vi "Labview_USB_GPIO_Test.vi"() -> ()   [LabVIEW 2012]
uses:
  Ginkgo PWM/Labview_USB_PWM_Test/lib/labview_32bit/ControlGPIO/Ginkgo_Driver.dll
panel:
  out "error out":errorcluster
  in  "stop":bool
  out "P8":bool
  out "P9":bool
  out "P10":bool
  out "P11":bool
  out "P12":bool
  out "P13":bool
  out "P14":bool
  out "P15":bool
  in  "P7":bool
  in  "P6":bool
  in  "P5":bool
  in  "P4":bool
  in  "P3":bool
  in  "P2":bool
  in  "P1":bool
  in  "P0":bool
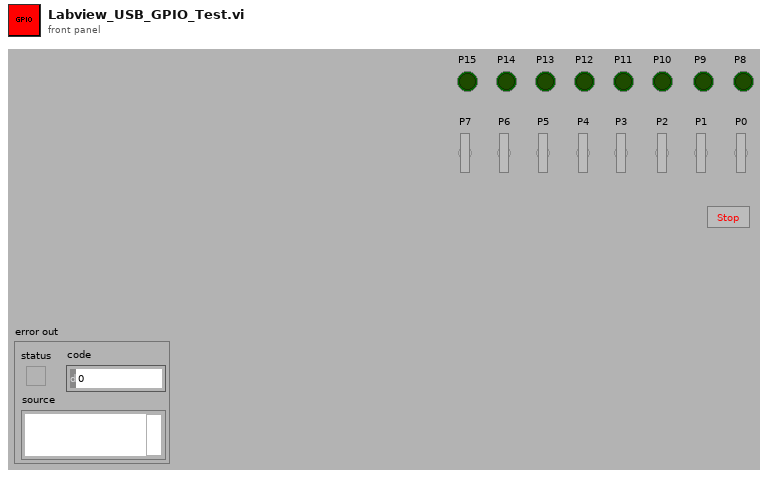
[diagram p1: front panel]
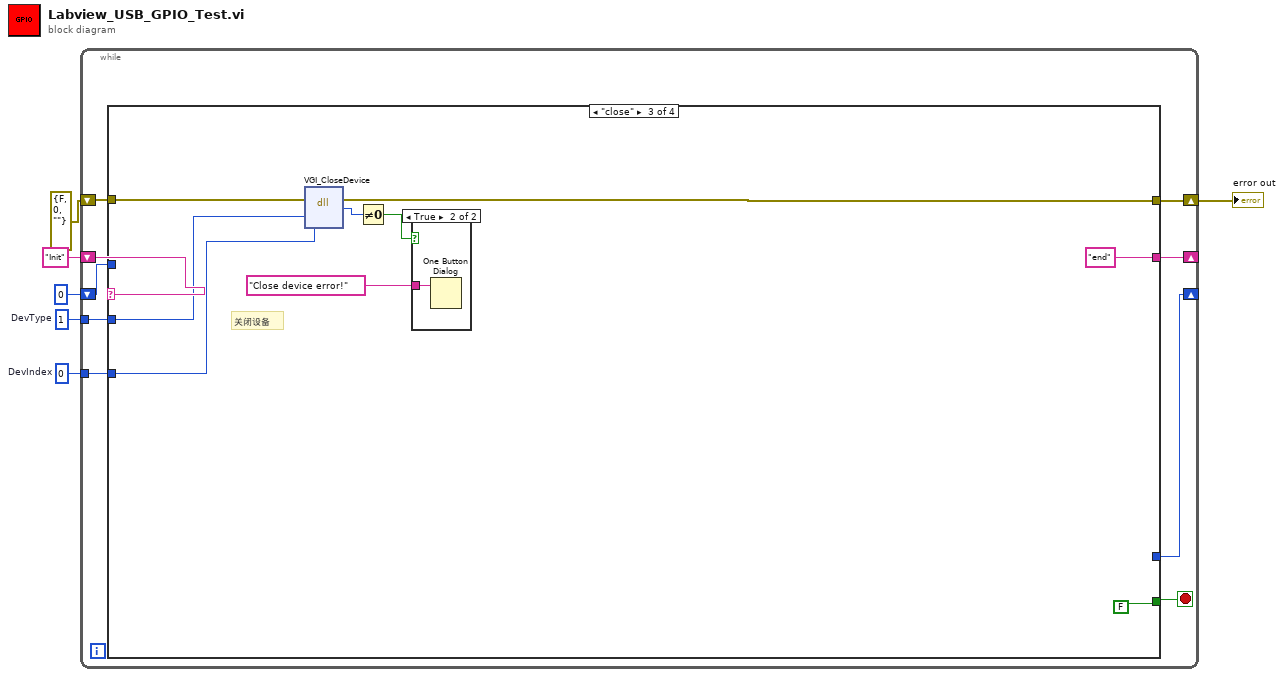
[diagram p0: block diagram]
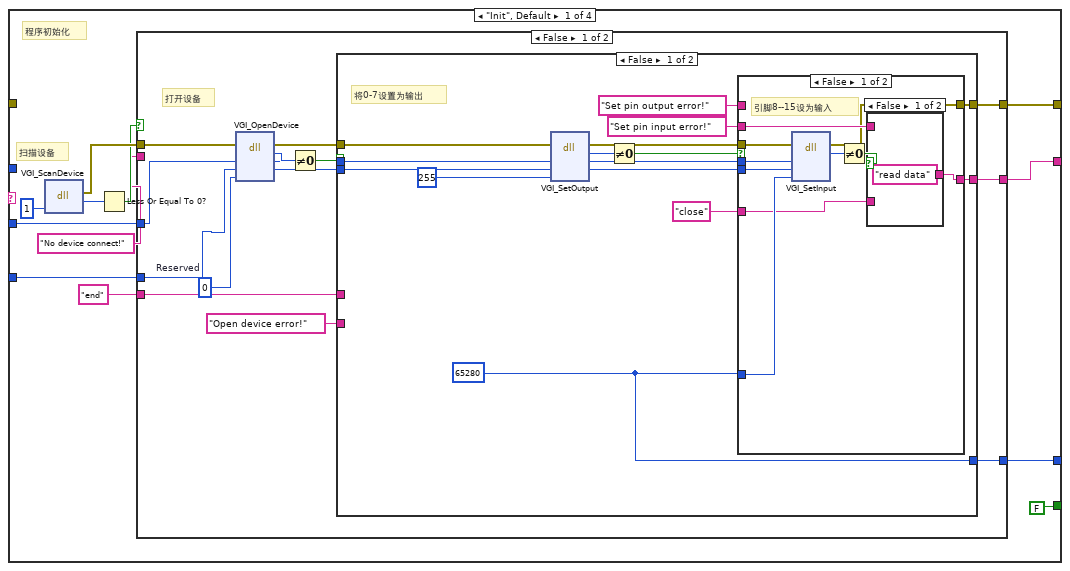
[diagram p2: hidden frame]
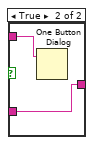
[diagram p3: hidden frame]
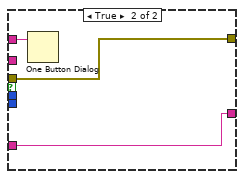
[diagram p4: hidden frame]
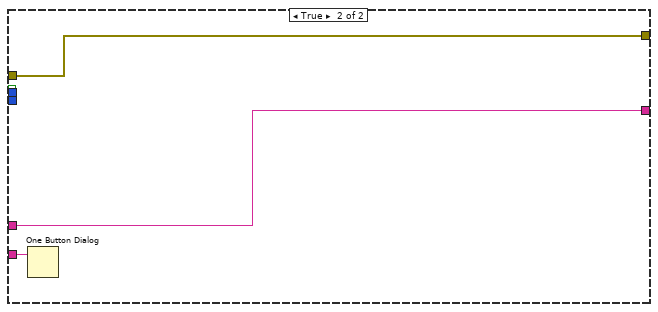
[diagram p5: hidden frame]
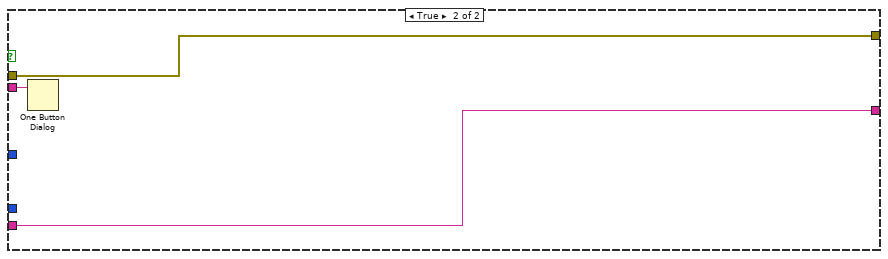
[diagram p6: hidden frame]
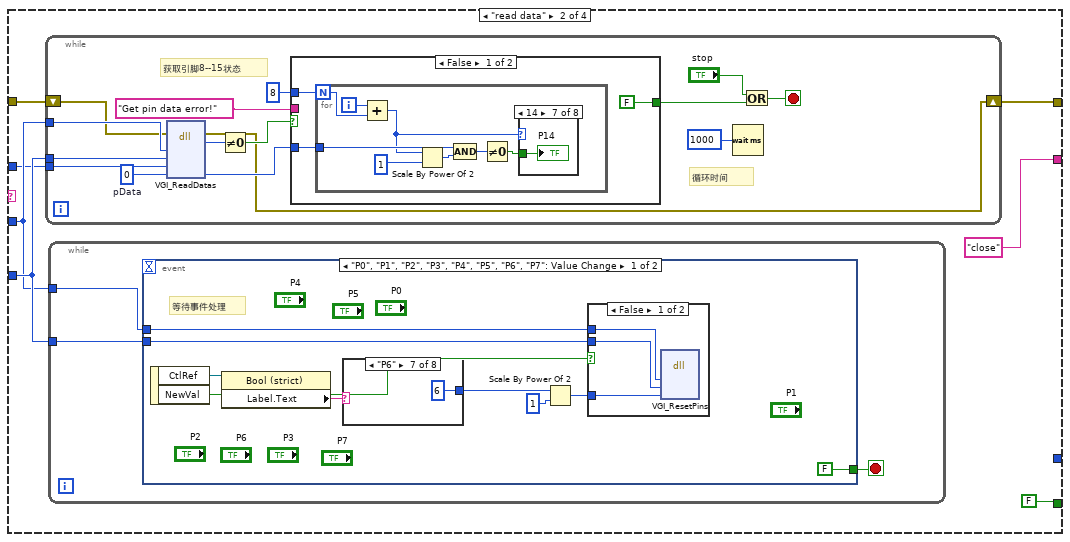
[diagram p7: hidden frame]
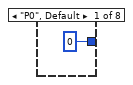
[diagram p8: hidden frame]
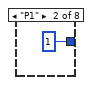
[diagram p9: hidden frame]
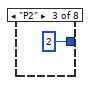
[diagram p10: hidden frame]
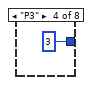
[diagram p11: hidden frame]
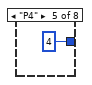
[diagram p12: hidden frame]
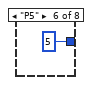
[diagram p13: hidden frame]
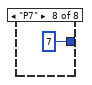
[diagram p14: hidden frame]
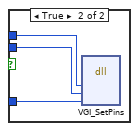
[diagram p15: hidden frame]
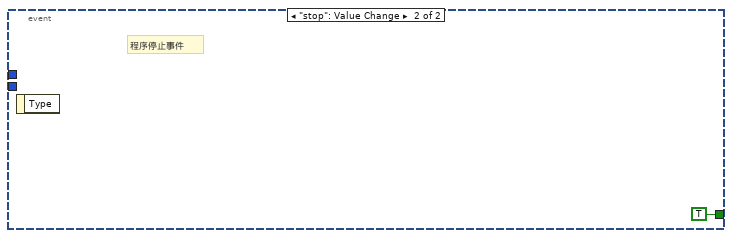
[diagram p16: hidden frame]
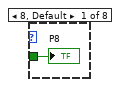
[diagram p17: hidden frame]
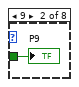
[diagram p18: hidden frame]
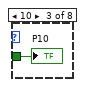
[diagram p19: hidden frame]
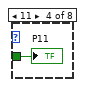
[diagram p20: hidden frame]
diagram:
  w4 = 0  # DevIndex
  w5 = 1  # DevType
  n1 = while {
    shift-right: [w14] -> _
    shift-left: "Init" -> [w15]
    tunnel: w5 -> [w13]
    tunnel: w4 -> [w12]
    shift-right: [w11] -> _
    shift-left: u16 0 -> [w10]
    shift-right: [w8] -> w2
    shift-left: errorcluster {"status"=FALSE, "code"=0, "source"=""} ("error out") -> [w7]
    stop <- w9 stop-if-true
    n2 = case shown="\"close\"" w15 {
      tunnel: [w21 "close" "end" "end"] -> w14
      tunnel: w13 -> [w20 w83 w149 _]
      tunnel: w12 -> [w19 w84 w150 _]
      tunnel: [w18 _ _ _] -> w11
      tunnel: w10 -> [_ w82 _ _]
      tunnel: [FALSE FALSE FALSE TRUE] -> w9
      tunnel: [w16 w79 w151 w159] -> w8
      tunnel: w7 -> [_ w80 w152 w159]
      frame "Init", Default {
        # "程序初始化"
        # "扫描设备"
        n3 = dll-call lib="E:/Project/vt_ginkgo/truck/Ginkgo Application Example/Labview/Ginkgo PWM/Labview_USB_PWM_Test/lib/labview_32bit/ControlGPIO/Ginkgo_Driver.dll" fn="VGI_ScanDevice"("NeedInit"=u8 1) -> (error out=w27:errorcluster, "return type"=w25:i32)  [unwired: 4 in, 1 out]
        n4 = Less Or Equal To 0?(x=w25) -> (x <= 0?=w24:bool)
        n5 = case shown="False" w24 {
          tunnel: "No device connect!" ("message") -> [_ w78]
          tunnel: w27 -> [w37 w76]
          tunnel: "end" -> [w35 w77]
          tunnel: [w34 w77] -> w21
          tunnel: w20 -> [w33 _]
          tunnel: w19 -> [w32 _]
          tunnel: [w29 _] -> w18
          tunnel: [w28 w76] -> w16
          frame False {
            w41 = 0  # Reserved
            # "打开设备"
            n6 = dll-call lib="E:/Project/vt_ginkgo/truck/Ginkgo Application Example/Labview/Ginkgo PWM/Labview_USB_PWM_Test/lib/labview_32bit/ControlGPIO/Ginkgo_Driver.dll" fn="VGI_OpenDevice"(error in=w37, "DevType"=w33, "DevIndex"=w32, "Reserved"=w41) -> (error out=w36:errorcluster, "return type"=w39:i32, "DevType"=w31:i32, "DevIndex"=w30:i32)  [unwired: 3 in, 1 out]
            n7 = Not Equal To 0?(x=w39) -> (x != 0?=w38:bool)
            n8 = case shown="False" w38 {
              tunnel: "Open device error!" ("message") -> [_ w75]
              tunnel: w36 -> [w53 w73]
              tunnel: w35 -> [_ w74]
              tunnel: [w52 w74] -> w34
              tunnel: w31 -> [w47 _]
              tunnel: w30 -> [w46 _]
              tunnel: [w43 _] -> w29
              tunnel: [w44 w73] -> w28
              frame False {
                w43 = u16 65280 ("y")
                # "将0-7设置为输出"
                n9 = dll-call lib="E:/Project/vt_ginkgo/truck/Ginkgo Application Example/Labview/Ginkgo PWM/Labview_USB_PWM_Test/lib/labview_32bit/ControlGPIO/Ginkgo_Driver.dll" fn="VGI_SetOutput"(error in=w53, "DevType"=w47, "DevIndex"=w46, "Pins"=u16 255) -> (error out=w49:errorcluster, "return type"=w55:i32, "DevType"=w50:i32, "DevIndex"=w51:i32)  [unwired: 3 in, 1 out]
                n10 = Not Equal To 0?(x=w55) -> (x != 0?=w56:bool)
                n11 = case shown="False" w56 {
                  tunnel: "Set pin output error!" ("message") -> [_ w72]
                  tunnel: [w59 w71] -> w52
                  tunnel: w43 -> [w66 _]
                  tunnel: w51 -> [w65 _]
                  tunnel: w50 -> [w64 _]
                  tunnel: w49 -> [w63 w70]
                  tunnel: "Set pin input error!" ("message") -> [w60 _]
                  tunnel: "close" -> [w58 w71]
                  tunnel: [w57 w70] -> w44
                  frame False {
                    # "引脚8--15设为输入"
                    n12 = dll-call lib="E:/Project/vt_ginkgo/truck/Ginkgo Application Example/Labview/Ginkgo PWM/Labview_USB_PWM_Test/lib/labview_32bit/ControlGPIO/Ginkgo_Driver.dll" fn="VGI_SetInput"(error in=w63, "DevType"=w64, "DevIndex"=w65, "Pins"=w66) -> (error out=w57:errorcluster, "return type"=w62:i32)  [unwired: 5 in, 1 out]
                    n13 = Not Equal To 0?(x=w62) -> (x != 0?=w61:bool)
                    n14 = case shown="False" w61 {
                      tunnel: w60 -> [_ w69]
                      tunnel: ["read data" w68] -> w59
                      tunnel: w58 -> [_ w68]
                      frame False {
                      }
                      frame True {
                        n15 = One Button Dialog(message=w69) -> ()  [unwired: 1 in, 1 out]
                      }
                    }
                  }
                  frame True {
                    n16 = One Button Dialog(message=w72) -> ()  [unwired: 1 in, 1 out]
                  }
                }
              }
              frame True {
                n17 = One Button Dialog(message=w75) -> ()  [unwired: 1 in, 1 out]
              }
            }
          }
          frame True {
            n18 = One Button Dialog(message=w78) -> ()  [unwired: 1 in, 1 out]
          }
        }
      }
      frame "read data" {
        n19 = while {
          tunnel: w83 -> [w118]
          tunnel: w84 -> [w117]
          tunnel: w82 -> [w116]
          shift-right: [w113] -> w79
          shift-left: w80 -> [w114]
          stop <- w119 stop-if-true
          w127 = u16 0  # pData
          # "获取引脚8--15状态"
          # "循环时间"
          n20 = dll-call lib="E:/Project/vt_ginkgo/truck/Ginkgo Application Example/Labview/Ginkgo PWM/Labview_USB_PWM_Test/lib/labview_32bit/ControlGPIO/Ginkgo_Driver.dll" fn="VGI_ReadDatas"(error in=w114, "DevType"=w118, "DevIndex"=w117, "PinMask"=w116, "pData"=w127) -> (error out=w113:errorcluster, "return type"=w126:i32, "pData"=w123:u16)  [unwired: 5 in, 1 out]
          n21 = Not Equal To 0?(x=w126) -> (x != 0?=w125:bool)
          n22 = case shown="False" w125 {
            tunnel: "Get pin data error!" ("message") -> [_ w148]
            tunnel: w123 -> [w130 _]
            tunnel: 8 -> [w129 _]
            tunnel: [FALSE TRUE] -> w120
            frame False {
              n23 = for {
                N: w129 -> [w133]
                tunnel: w130 -> [w135]
                i -> [w134]
                n24 = Add(x=w134, y=w133) -> (x+y=w132:i32)
                n25 = Scale By Power Of 2(n=w132, x=u16 1) -> (x*2^n=w136:u16)
                n26 = Compound Arithmetic op=AND(w135, w136) -> (w138:u16)
                n27 = Not Equal To 0?(x=w138) -> (x != 0?=w131:bool)
                n28 = case shown="14" w132 {
                  tunnel: w131 -> [w139 w140 w141 w142 w143 w144 w145 w146]
                  frame 8, Default {
                    "P8" <- w139
                  }
                  frame 9 {
                    "P9" <- w140
                  }
                  frame 10 {
                    "P10" <- w141
                  }
                  frame 11 {
                    "P11" <- w142
                  }
                  frame 12 {
                    "P12" <- w143
                  }
                  frame 13 {
                    "P13" <- w144
                  }
                  frame 14 {
                    "P14" <- w145
                  }
                  frame 15 {
                    "P15" <- w146
                  }
                }
              }
            }
            frame True {
              n29 = One Button Dialog(message=w148) -> ()  [unwired: 1 in, 1 out]
            }
          }
          n30 = Wait (ms)(milliseconds to wait=u32 1000) -> ()  [unwired: 1 out]
          n31 = Or(x="stop", y=w120) -> (x .or. y?=w119:bool)
        }
        n32 = while {
          tunnel: w84 -> [w87]
          tunnel: w83 -> [w86]
          stop <- w88 stop-if-true
          n33 = event shown="[0] \"P0\", \"P1\", \"P2\", \"P3\", \"P4\", \"P5\", \"P6\", \"P7\": Value Change" {
            selector: _ -> [_ _]
            dyn-events: _ -> [_ _]
            timeout: _ -> [_ _]
            tunnel: [FALSE ("stop") TRUE ("stop")] -> w88
            tunnel: w86 -> [w94 _]
            tunnel: w87 -> [w93 _]
            event "P0", "P1", "P2", "P3", "P4", "P5", "P6", "P7": Value Change {
              # "等待事件处理"
              n34 = event-data() -> ("CtlRef"=w96:refnum<vi>, "NewVal"=w95:bool)  [unwired: 1 in]
              n35 = property class="Bool (strict)"(reference=w96) -> ("Label.Text"=w90:string)  [unwired: 1 in, 2 out]
              n36 = case shown="\"P6\"" w90 {
                tunnel: [0 1 2 3 4 5 6 7] -> w89
                frame "P0", Default {
                }
                frame "P1" {
                }
                frame "P2" {
                }
                frame "P3" {
                }
                frame "P4" {
                }
                frame "P5" {
                }
                frame "P6" {
                }
                frame "P7" {
                }
              }
              n37 = Scale By Power Of 2(n=w89, x=u16 1) -> (x*2^n=w91:u16)
              n38 = case shown="False" w95 {
                tunnel: w94 -> [w108 w111]
                tunnel: w93 -> [w107 w110]
                tunnel: w91 -> [w106 w109]
                frame False {
                  n39 = dll-call lib="E:/Project/vt_ginkgo/truck/Ginkgo Application Example/Labview/Ginkgo PWM/Labview_USB_PWM_Test/lib/labview_32bit/ControlGPIO/Ginkgo_Driver.dll" fn="VGI_ResetPins"("DevType"=w108, "DevIndex"=w107, "Pins"=w106) -> ()  [unwired: 7 in, 2 out]
                }
                frame True {
                  n40 = dll-call lib="E:/Project/vt_ginkgo/truck/Ginkgo Application Example/Labview/Ginkgo PWM/Labview_USB_PWM_Test/lib/labview_32bit/ControlGPIO/Ginkgo_Driver.dll" fn="VGI_SetPins"("DevType"=w111, "DevIndex"=w110, "Pins"=w109) -> ()  [unwired: 7 in, 2 out]
                }
              }
            }
            event "stop": Value Change {
              # "程序停止事件"
              n41 = event-data() -> ()  [unwired: 1 in, 1 out]
            }
          }
        }
      }
      frame "close" {
        # "关闭设备"
        n42 = dll-call lib="E:/Project/vt_ginkgo/truck/Ginkgo Application Example/Labview/Ginkgo PWM/Labview_USB_PWM_Test/lib/labview_32bit/ControlGPIO/Ginkgo_Driver.dll" fn="VGI_CloseDevice"(error in=w152, "DevType"=w149, "DevIndex"=w150) -> (error out=w151:errorcluster, "return type"=w155:i32)  [unwired: 4 in, 1 out]
        n43 = Not Equal To 0?(x=w155) -> (x != 0?=w157:bool)
        n44 = case shown="True" w157 {
          tunnel: "Close device error!" ("message") -> [_ w158]
          frame False {
          }
          frame True {
            n45 = One Button Dialog(message=w158) -> ()  [unwired: 1 in, 1 out]
          }
        }
      }
      frame "end" {
      }
    }
  }
  "error out" <- w2
